vi "CF_TC_to_DSC.vi"(2 "dbl":dbl[](array[numeric]), 3 "dbl var":refnum<k21>[](array[refnum])=["ni.var.psp://housesoftheholy/Leiden CF900/Leiden CF TC/CF TC R0", "ni.var.psp://housesoftheholy/Leiden CF900/Leiden CF TC/CF TC R1", "ni.var.psp://housesoftheholy/Leiden CF900/Leiden CF TC/CF TC R2", "ni.var.psp://housesoftheholy/Leiden CF900/Leiden CF TC/CF TC R3", "ni.var.psp://housesoftheholy/Leiden CF900/Leiden CF TC/CF TC R4", "ni.var.psp://housesoftheholy/Leiden CF900/Leiden CF TC/CF TC R5", "ni.var.psp://housesoftheholy/Leiden CF900/Leiden CF TC/CF TC R6", "ni.var.psp://housesoftheholy/Leiden CF900/Leiden CF TC/CF TC R7", "ni.var.psp://housesoftheholy/Leiden CF900/Leiden CF TC/CF TC T0", "ni.var.psp://housesoftheholy/Leiden CF900/Leiden CF TC/CF TC T1", "ni.var.psp://housesoftheholy/Leiden CF900/Leiden CF TC/CF TC T2", "ni.var.psp://housesoftheholy/Leiden CF900/Leiden CF TC/CF TC T3", "ni.var.psp://housesoftheholy/Leiden CF900/Leiden CF TC/CF TC T4", "ni.var.psp://housesoftheholy/Leiden CF900/Leiden CF TC/CF TC T5", "ni.var.psp://housesoftheholy/Leiden CF900/Leiden CF TC/CF TC T6", "ni.var.psp://housesoftheholy/Leiden CF900/Leiden CF TC/CF TC T7", "ni.var.psp://housesoftheholy/Leiden CF900/Leiden CF TC/CF TC I0", "ni.var.psp://housesoftheholy/Leiden CF900/Leiden CF TC/CF TC I1", "ni.var.psp://housesoftheholy/Leiden CF900/Leiden CF TC/CF TC I2", "ni.var.psp://housesoftheholy/Leiden CF900/Leiden CF TC/CF TC I3"]) -> ()   [LabVIEW 2013]
panel:
  # "CF TC to DSC"
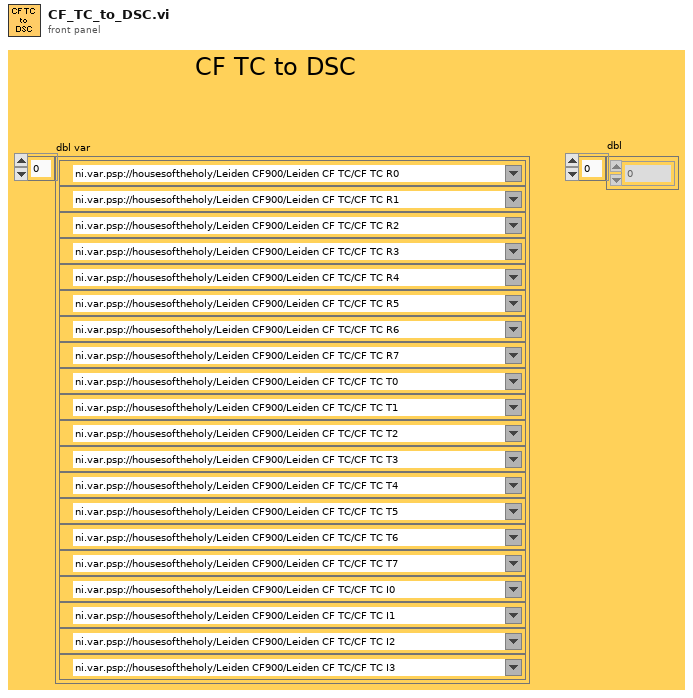
[diagram p1: front panel]
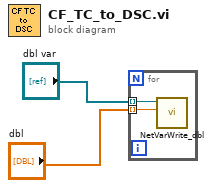
[diagram p0: block diagram]
diagram:
  n1 = for {
    tunnel: "dbl var" -> [w4] mode=indexing
    tunnel: "dbl" -> [w3] mode=indexing
    n2 = call "NetVarWrite_dbl.vi"("Numeric"=w3, "Refnum in"=w4) -> ()  [unwired: 10 in]
  }
